vi "Log Assert Core.vi"   [LabVIEW 2016, in "AssertEngine.lvlib"]
uses:
  AssertEngine.lvlib
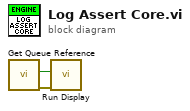
[diagram p0: block diagram]
diagram:
  n1 = call "Get Queue Reference.vi"() -> ("error out"=w1:errorcluster, "created new?"=w2:bool)  [unwired: 9 in, 1 out]
  n2 = call "Run Display.vi"("error in (no error)"=w1, "Run?"=w2) -> ()  [unwired: 9 in, 1 out]
